vi "ep_Zoom FFT (1 Channel).vi"(0 "signal":dbl[](array[numeric]) format="%.2f", 1 "phase output? (F)":bool, 2 "reset? (F)":bool, 5 "zoom FFT settings":T2 {"FFT settings"."window" items=["Rectangle"=0, "Hanning"=1, "Hamming"=2, "Blackman-Harris"=3, "Exact Blackman"=4, "Blackman"=5, "Flat Top"=6, "4 Term B-Harris "=7, "7 Term B-Harris"=8, "Low Sidelobe"=9, "Blackman Nuttall"=11, "Triangle"=30, "Bartlett-Hanning"=31, "Bohman"=32, "Parzen"=33, "Welch"=34, "Kaiser"=60, "Dolph-Chebyshev"=61, "Gaussian"=62]}, 9 "dB on? (T)":bool=TRUE, 11 "error in (no error)":errorcluster, 12 "zoom FFT state in":T1, 13 "demodulated? (F)":bool) -> (4 "FFT magnitude":cluster{"f0":dbl, "df":dbl, "magnitude":dbl[]}, 6 "FFT phase":cluster{"f0":dbl, "df":dbl, "phase":dbl[]}, 10 "spectrum ready?":bool, 14 "zoom FFT state out":T1, 15 "error out":errorcluster)   [LabVIEW 2014, in "NI_EP_Motor Monitoring.lvlib"]
uses:
  <vilib>/addons/Electrical Power/Motor Monitoring/NI_EP_Motor Monitoring.lvlib
  <vilib>/addons/Electrical Power/Motor Monitoring/subVIs/ep_Zoom FFT Settings.ctl
  <vilib>/Analysis/NI_AALPro.lvlib
  <vilib>/measure/NI_MAPro.lvlib
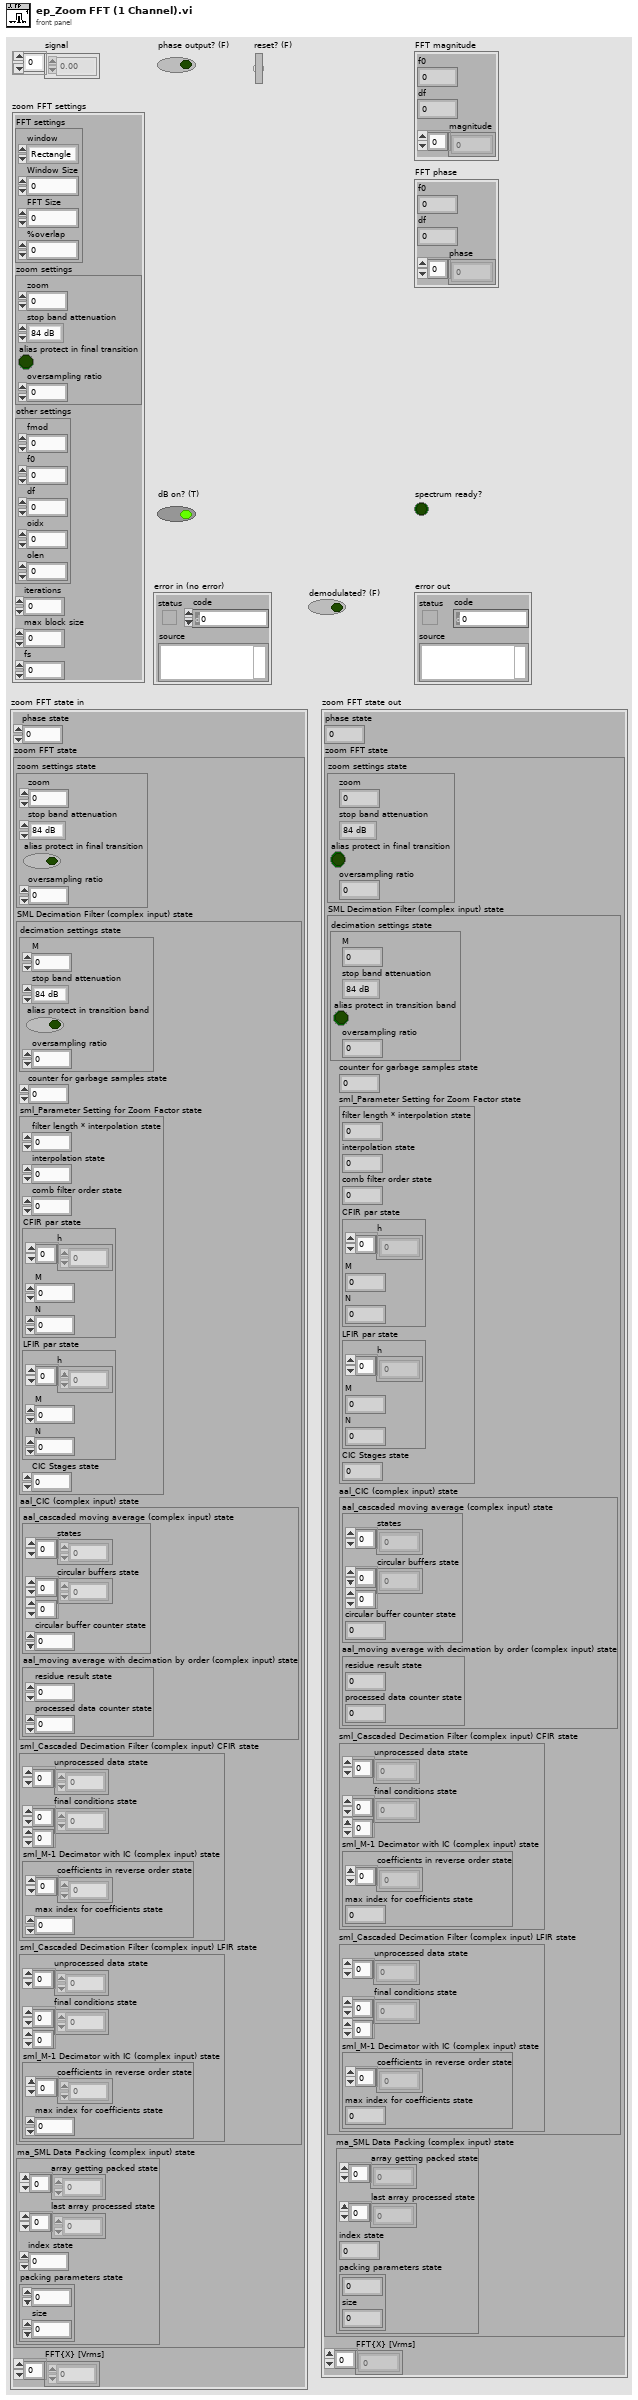
[diagram p1: front panel]
types:
  T1 = cluster{"phase state":dbl, "zoom FFT state":cluster{"zoom settings state":cluster{"zoom":i32, "stop band attenuation":enum16{"84 dB", "96 dB", "120 dB"}, "alias protect in final transition":bool, "oversampling ratio":dbl}, "SML Decimation Filter (complex input) state":cluster{"decimation settings state":cluster{"M":i32, "stop band attenuation":enum16{"84 dB", "96 dB", "120 dB"}, "alias protect in transition band":bool, "oversampling ratio":dbl}, "counter for garbage samples state":i32, "sml_Parameter Setting for Zoom Factor state":cluster{"filter length * interpolation state":i32, "interpolation state":i32, "comb filter order state":i32, "CFIR par state":cluster{"h":dbl[], "M":i32, "N":i32}, "LFIR par state":cluster{"h":dbl[], "M":i32, "N":i32}, "CIC Stages state":i32}, "aal_CIC (complex input) state":cluster{"aal_cascaded moving average (complex input) state":cluster{"states":cdb[], "circular buffers state":cdb[][], "circular buffer counter state":i32}, "aal_moving average with decimation by order (complex input) state":cluster{"residue result state":cdb, "processed data counter state":i32}}, "sml_Cascaded Decimation Filter (complex input) CFIR state":cluster{"unprocessed data state":cdb[], "final conditions state":cdb[][], "sml_M-1 Decimator with IC (complex input) state":cluster{"coefficients in reverse order state":dbl[], "max index for coefficients state":i32}}, "sml_Cascaded Decimation Filter (complex input) LFIR state":cluster{"unprocessed data state":cdb[], "final conditions state":cdb[][], "sml_M-1 Decimator with IC (complex input) state":cluster{"coefficients in reverse order state":dbl[], "max index for coefficients state":i32}}}, "ma_SML Data Packing (complex input) state":cluster{"array getting packed state":cdb[], "last array processed state":cdb[], "index state":i32, "packing parameters state":cluster{i32, "size":i32}}}, "FFT{X} [Vrms]":cdb[]}
  T2 = typedef "NI_EP_Motor Monitoring.lvlib/ep_Zoom FFT Settings.ctl" = cluster{"FFT settings":cluster{"window":u16, "Window Size":i32, "FFT Size":i32, "%overlap":dbl}, "zoom settings":cluster{"zoom":i32, "stop band attenuation":enum16{"84 dB", "96 dB", "120 dB"}, "alias protect in final transition":bool, "oversampling ratio":dbl}, "other settings":cluster{"fmod":dbl, "f0":dbl, "df":dbl, "oidx":i32, "olen":i32}, "iterations":i32, "max block size":i32, "fs":dbl}
  T3 = cluster{"zoom":i32, "stop band attenuation":enum16{"84 dB", "96 dB", "120 dB"}, "alias protect in final transition":bool, "oversampling ratio":dbl}
  T4 = cluster{"window":u16, "Window Size":i32, "FFT Size":i32, "%overlap":dbl}
  T5 = cluster{"zoom settings state":cluster{"zoom":i32, "stop band attenuation":enum16{"84 dB", "96 dB", "120 dB"}, "alias protect in final transition":bool, "oversampling ratio":dbl}, "SML Decimation Filter (complex input) state":cluster{"decimation settings state":cluster{"M":i32, "stop band attenuation":enum16{"84 dB", "96 dB", "120 dB"}, "alias protect in transition band":bool, "oversampling ratio":dbl}, "counter for garbage samples state":i32, "sml_Parameter Setting for Zoom Factor state":cluster{"filter length * interpolation state":i32, "interpolation state":i32, "comb filter order state":i32, "CFIR par state":cluster{"h":dbl[], "M":i32, "N":i32}, "LFIR par state":cluster{"h":dbl[], "M":i32, "N":i32}, "CIC Stages state":i32}, "aal_CIC (complex input) state":cluster{"aal_cascaded moving average (complex input) state":cluster{"states":cdb[], "circular buffers state":cdb[][], "circular buffer counter state":i32}, "aal_moving average with decimation by order (complex input) state":cluster{"residue result state":cdb, "processed data counter state":i32}}, "sml_Cascaded Decimation Filter (complex input) CFIR state":cluster{"unprocessed data state":cdb[], "final conditions state":cdb[][], "sml_M-1 Decimator with IC (complex input) state":cluster{"coefficients in reverse order state":dbl[], "max index for coefficients state":i32}}, "sml_Cascaded Decimation Filter (complex input) LFIR state":cluster{"unprocessed data state":cdb[], "final conditions state":cdb[][], "sml_M-1 Decimator with IC (complex input) state":cluster{"coefficients in reverse order state":dbl[], "max index for coefficients state":i32}}}, "ma_SML Data Packing (complex input) state":cluster{"array getting packed state":cdb[], "last array processed state":cdb[], "index state":i32, "packing parameters state":cluster{i32, "size":i32}}}
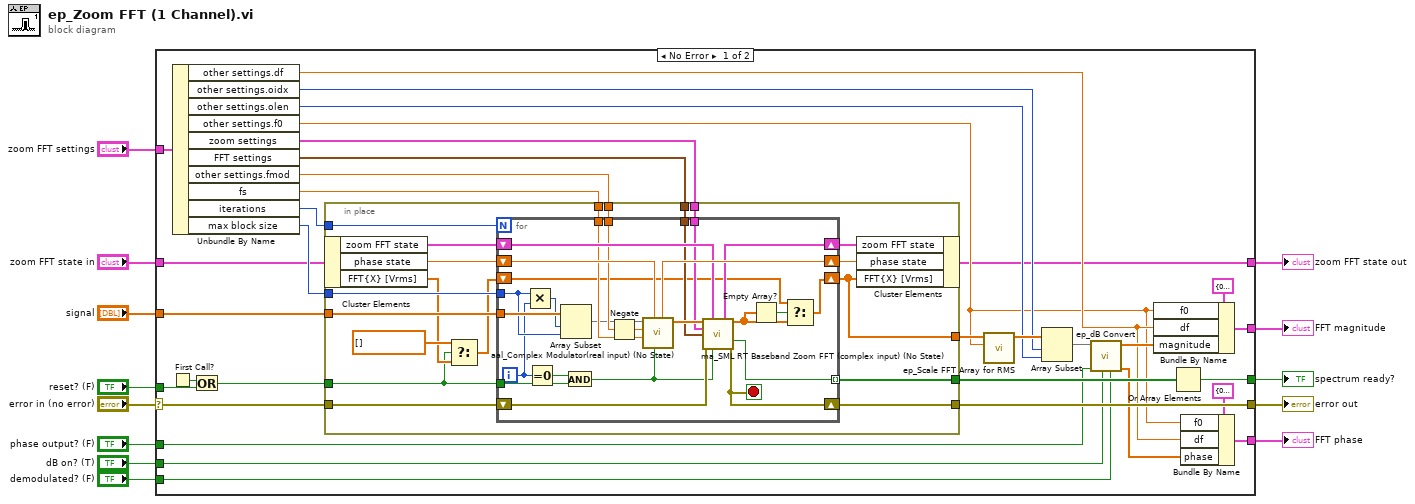
[diagram p0: block diagram]
diagram:
  n1 = case shown="No Error" "error in (no error)" {
    selector: "error in (no error)" -> [w45 w91]
    tunnel: [w37 _] -> w13
    tunnel: "signal" -> [w46 _]
    tunnel: [w28 _] -> w10
    tunnel: [w44 w91] -> w9
    tunnel: "reset? (F)" -> [w25 _]
    tunnel: "zoom FFT settings" -> [w42 _]
    tunnel: "dB on? (T)" -> [w30 _]
    tunnel: "demodulated? (F)" -> [w29 _]
    tunnel: "zoom FFT state in" -> [w16 _]
    tunnel: [w14 _] -> w3
    tunnel: "phase output? (F)" -> [w23 _]
    tunnel: [w22 _] -> w1
    frame No Error {
      n2 = First Call?() -> (First Call?: T/F=w24:bool)
      n3 = Unbundle By Name(w42) -> ("other settings.df"=w19:dbl, "other settings.oidx"=w31:i32, "other settings.olen"=w32:i32, "other settings.f0"=w18:dbl, "zoom settings"=w38:T3, "FFT settings"=w39:T4, "other settings.fmod"=w40:dbl, "fs"=w41:dbl, "iterations"=w15:i32, "max block size"=w36:i32)
      n4 = Or(x=w24, y=w25) -> (x .or. y?=w26:bool)
      n5 = in-place {
        in-place-border: w46 -> [w65]
        in-place-border: w45 -> [w64]
        in-place-border: [w63] -> w44
        in-place-border: [w62] -> w43
        in-place-border: w41 -> [w61]
        in-place-border: w40 -> [w60]
        in-place-border: w39 -> [w59]
        in-place-border: w38 -> [w58]
        in-place-border: w15 -> [w57]
        in-place-border: w36 -> [w56]
        in-place-border: [w50] -> w27
        in-place-border: w26 -> [w51]
        n6 = in-place-cluster #1(w16) -> ("zoom FFT state"=w55:T5, "phase state"=w54:dbl, "FFT{X} [Vrms]"=w52:cdb[])
        n7 = Select(t=cdb[] [], s=w51, f=w52) -> (s? t:f=w47:cdb[])
        n8 = for {
          N: w57 -> [_]
          tunnel: w65 -> [w78]
          tunnel: w51 -> [w72]
          tunnel: [w87] -> w62 mode=indexing
          tunnel: w61 -> [w82]
          tunnel: w60 -> [w81]
          tunnel: w59 -> [w80]
          tunnel: w58 -> [w79]
          shift-right: [w85] -> w49
          shift-left: w54 -> [w86]
          shift-right: [w83] -> w48
          shift-left: w55 -> [w84]
          shift-right: [w66] -> w63
          shift-left: w64 -> [w88]
          tunnel: w56 -> [w75]
          shift-right: [w68] -> w50
          shift-left: w47 -> [w67]
          i -> [w74]
          stop <- w66 stop-if-true
          n9 = Multiply(x=w75, y=w74) -> (x*y=w76:i32)
          n10 = Equal To 0?(x=w74) -> (x = 0?=w73:bool)
          n11 = Array Subset(array=w78, index=w76, length=w75) -> (w77:dbl[])
          n12 = And(x=w73, y=w72) -> (x .and. y?=w71:bool)
          n13 = Negate(x=w81) -> (-x=w90:dbl)
          n14 = call <vilib>:"aal_Complex Modulator(real input) (No State).vi"("reset ?"=w71, "initial phase"=w86, "fs"=w82, "frequency"=w90, "x"=w77) -> ("y"=w89:cdb[], "next initial phase"=w85:dbl)  [unwired: 5 in]
          n15 = call <vilib>:"ma_SML RT Baseband Zoom FFT (complex input) (No State).vi"("x [V]"=w89, "SML RT Baseband Zoom FFT (complex input) state in"=w84, "zoom settings"=w79, "FFT settings"=w80, "error in (no error)"=w88, "reset?"=w71) -> ("SML RT Baseband Zoom FFT (complex input) state out"=w83:T5, "FFT{X} [Vrms]"=w69:cdb[], "spectrum ready?"=w87:bool, "error out"=w66:errorcluster)  [unwired: 3 in, 3 out]
          n16 = Empty Array?(array=w69) -> (empty?=w70:bool)
          n17 = Select(t=w67, s=w70, f=w69) -> (s? t:f=w68:cdb[])
        }
        n18 = in-place-cluster #1("zoom FFT state"=w48, "phase state"=w49, "FFT{X} [Vrms]"=w50) -> (w14:T1)
      }
      n19 = call <vilib>:"ep_Scale FFT Array for RMS.vi"("f0"=w18, "FFT{X} [EU]"=w27) -> ("FFT {X} [rms]"=w35:cdb[])  [unwired: 9 in]
      n20 = Array Subset(array=w35, index=w31, length=w32) -> (w34:cdb[])
      n21 = call <vilib>:"ep_dB Convert.vi"("demodulated? (F)"=w29, "dB on? (T)"=w30, "phase output? (F)"=w23, "spectrum in"=w34) -> ("phase"=w20:dbl[], "magnitude"=w33:dbl[])  [unwired: 6 in]
      n22 = Bundle By Name(cluster=cluster{"f0":dbl, "df":dbl, "magnitude":dbl[]} {"f0"=0.0, "df"=0.0, "magnitude"=[]} ("FFT magnitude"), "f0"=w18, "df"=w19, "magnitude"=w33) -> (w28:cluster{"f0":dbl, "df":dbl, "magnitude":dbl[]})
      n23 = Or Array Elements(Boolean array=w43) -> (logical OR=w37:bool)
      n24 = Bundle By Name(cluster=cluster{"f0":dbl, "df":dbl, "phase":dbl[]} {"f0"=0.0, "df"=0.0, "phase"=[]} ("FFT phase"), "f0"=w18, "df"=w19, "phase"=w20) -> (w22:cluster{"f0":dbl, "df":dbl, "phase":dbl[]})
    }
    frame Error {
    }
  }
  "spectrum ready?" <- w13
  "FFT magnitude" <- w10
  "error out" <- w9
  "zoom FFT state out" <- w3
  "FFT phase" <- w1
